vi "LVClass_ClosedLoopSecurityActivation_Ctor.vi"(0 "ClosedLoopSecurity (const)":refnum<class "ClosedLoopSecurityActivation.lvclass">, 5 "ClosedLoopSecurityParams":T1, 11 "error in (no error)":errorcluster) -> (4 "ClosedLoopSecurity (new)":refnum<class "ClosedLoopSecurityActivation.lvclass">, 15 "error out":errorcluster)   [LabVIEW 2020, in "ClosedLoopSecurityActivation.lvclass"]
doc: "Manual construction.\n\n<B>security_activationIn</B> : Constant Pointer to Closed Loop security activation object.\n<B>security_activationOut</B> : Constant Pointer to Closed Loop security activation object.\n<B>do_check_saturated_act_count</B> : Activates the requested actuators positions check, test will return false if\n too many acturators reach their boundaries\n<B>do_check_camera_fill_pct</B> : Activates the camera saturation level check\n<B>do_check_pupil_size_variation</B> : Activates the pupil size variation check, test will return false if pupil is\n too different from the interaction matrix pupil\n<B>do_check_dwf_pv</B> : Activates the delta wavefront peak-to-valley check"
uses:
  ClosedLoopSecurityActivation.lvclass
  Controls/ClosedLoopSecurityActivationParameters.ctl
  Controls/Handle creation.ctl
  ClosedLoopSecurityActivation.lvclass/ClosedLoopSecurityActivation.ctl
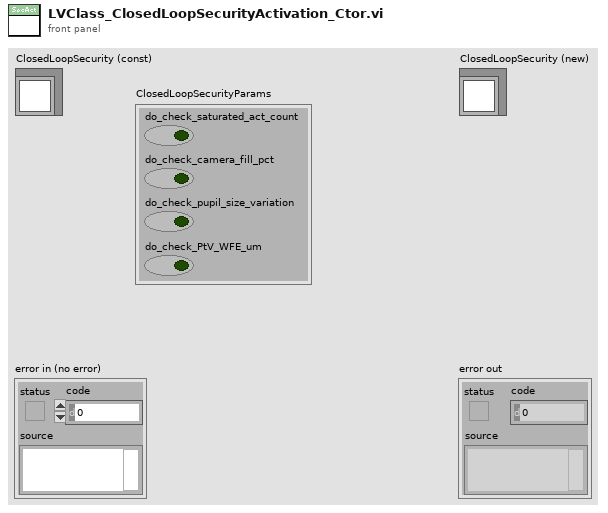
[diagram p1: front panel]
types:
  T1 = typedef "ClosedLoopSecurityActivationParameters.ctl" = cluster{"do_check_saturated_act_count":bool, "do_check_camera_fill_pct":bool, "do_check_pupil_size_variation":bool, "do_check_PtV_WFE_um":bool}
  T2 = typedef "Handle creation.ctl" = enum16{"By ctor", "By write function"}
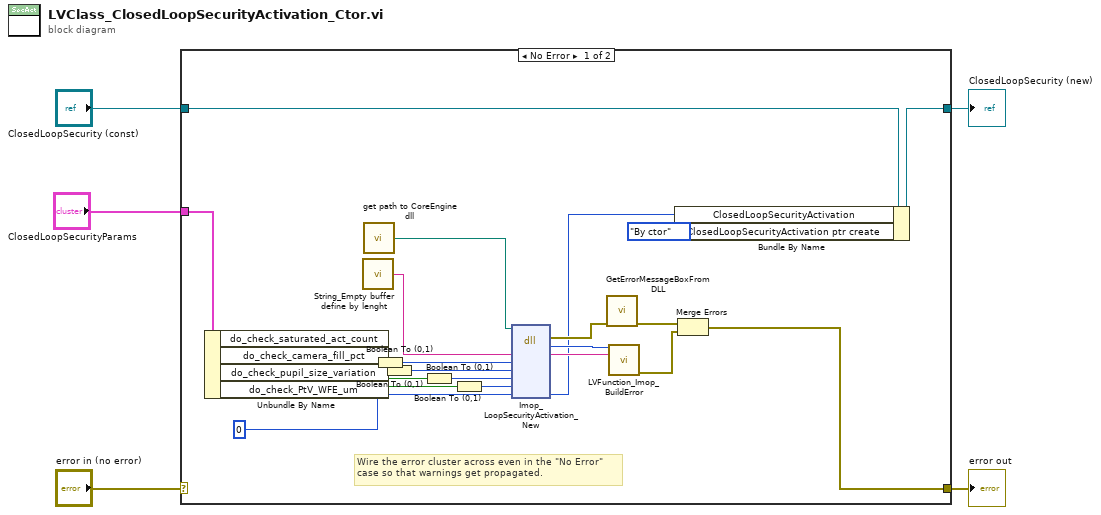
[diagram p0: block diagram]
diagram:
  n1 = case shown="No Error" "error in (no error)" {
    selector: "error in (no error)" -> [_ w29]
    tunnel: [w15 w29] -> w4
    tunnel: [w16 w28] -> w2
    tunnel: "ClosedLoopSecurity (const)" -> [w17 w28]
    tunnel: "ClosedLoopSecurityParams" -> [w14 _]
    frame No Error {
      # "Wire the error cluster across even in the \"No Error\"\ncase so that warnings get propagated."
      n2 = Unbundle By Name(w14) -> ("do_check_saturated_act_count"=w13:bool, "do_check_camera_fill_pct"=w12:bool, "do_check_pupil_size_variation"=w11:bool, "do_check_PtV_WFE_um"=w10:bool)
      n3 = call "String_Empty buffer define by lenght.vi"() -> ("Empty buffer"=w27:string)  [unwired: 1 in]
      n4 = call "get path to CoreEngine dll.vi"() -> ("path to wavekit library"=w18:path)  [unwired: 14 in, 1 out]
      n5 = Boolean To (0,1)(Boolean=w13) -> (0, 1=w9:i16)
      n6 = Boolean To (0,1)(Boolean=w12) -> (0, 1=w8:i16)
      n7 = Boolean To (0,1)(Boolean=w11) -> (0, 1=w7:i16)
      n8 = Boolean To (0,1)(Boolean=w10) -> (0, 1=w6:i16)
      n9 = dll-call lib="D:/soft/HASO_v3/SVN_trunk/ImOpCoreEngine4_LV2011/DLLs/c_interface_vc100.dll" fn="Imop_LoopSecurityActivation_New"(path in=w18, "message"=w27, "do_check_saturated_act_count"=w9, "do_check_camera_fill_pct"=w8, "do_check_pupil_size_variation"=w7, "do_check_loop_gain"=w6, "security_activation"=0 ("Pupil")) -> (error out=w24:errorcluster, "return type"=w25:i32, "message"=w26:string, "security_activation"=w22:i64)  [unwired: 6 in, 1 out]
      n10 = call "GetErrorMessageBoxFromDLL.vi"("error IN"=w24) -> ("error OUT"=w20:errorcluster)  [unwired: 10 in]
      n11 = call "LVFunction_Imop_BuildError.vi"("code"=w25, "String to Prepend to source (\"\")"=w26) -> ("error out"=w19:errorcluster)  [unwired: 13 in]
      n12 = Bundle By Name(cluster=w17, "ClosedLoopSecurityActivation"=w22, "ClosedLoopSecurityActivation ptr create"=Handle_creation."By ctor" ("Pupil ptr create")) -> (w16:refnum<class "ClosedLoopSecurityActivation.lvclass">)
      n13 = Merge Errors(w20, w19) -> (w15:errorcluster)
    }
    frame Error {
    }
  }
  "error out" <- w4
  "ClosedLoopSecurity (new)" <- w2
